vi "main_WS.vi"() -> ()   [LabVIEW 2017]
uses:
  <vilib>/Instr/_visa.llb/VISA Configure Serial Port (Instr).vi
panel:
  out "Waveform Chart":dbl(graph)
  in  "Reconnect":bool
  out "read buffer":string
  in  "Exit":bool
  in  "baud rate":u32=57600
  in  "VISA resource name":refnum<visa-resource-name>="COM1"
  out "tVOC":dbl
  out "CO2":dbl
  out "altitude":dbl
  in  "altitude2":dbl(slide) caption="m" scale=0.0..1000.0 scale format="%#_6p"
  in  "humidity2":dbl(slide) caption="%" scale=0.0..100.0 scale format="%#_6p"
  in  "temperature2":dbl(slide) caption="°C" scale=-20.0..100.0 scale format="%#_6p"
  in  "pressure2":dbl(slide) caption="Pa" scale=110.0..110000.0 scale format="%#_6p"
  out "Humidity":dbl
  out "temperature":dbl
  out "pressure":dbl
  # "Weather Station"
  # "Pressure"
  # "Humidity"
  # "Temperature"
  # "Altitude"
  # "Air quality"
  # "Communication:"
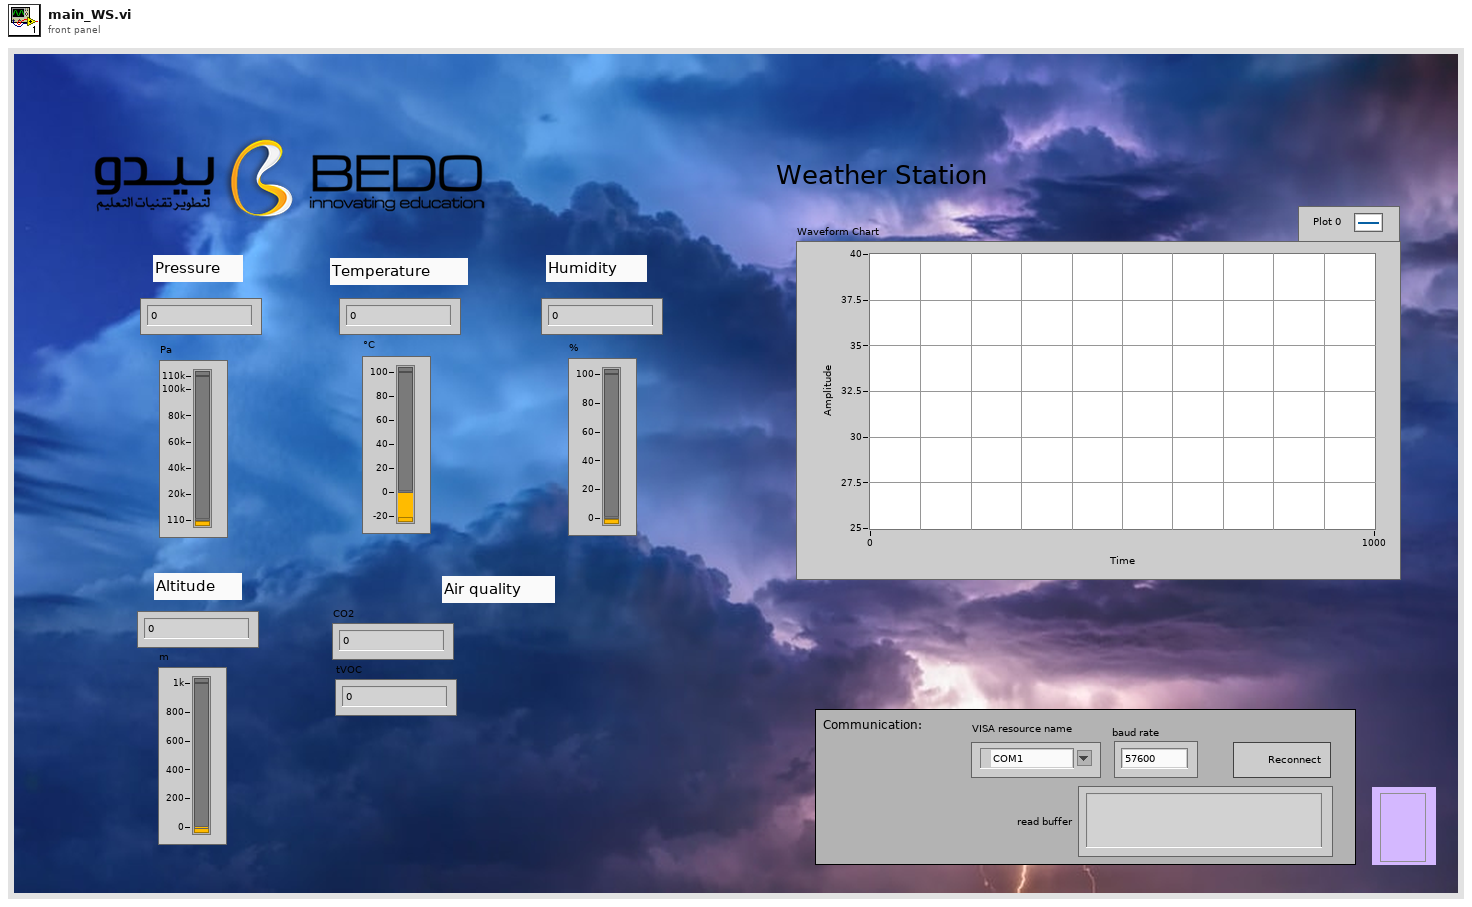
[diagram p1: front panel]
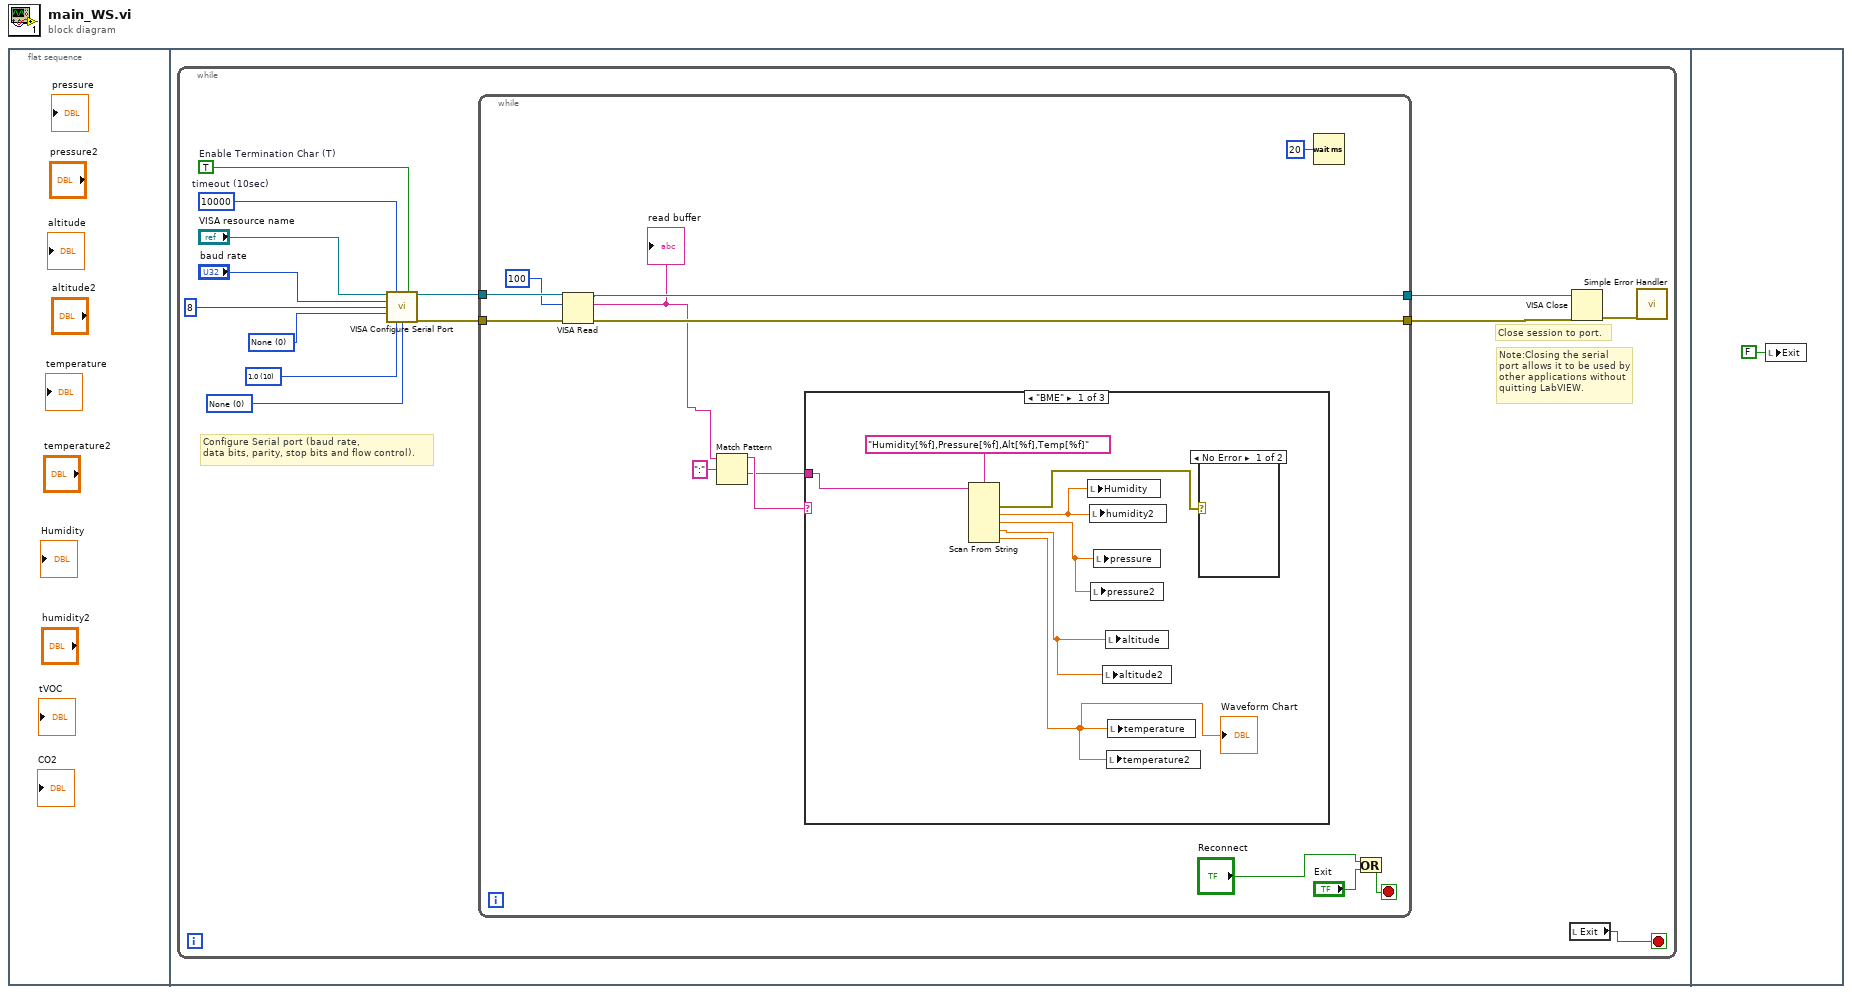
[diagram p0: block diagram]
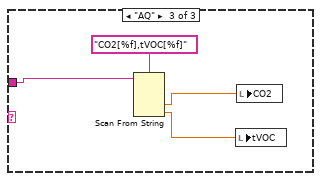
[diagram p4: hidden frame]
diagram:
  n1 = flat-sequence {
    frame #0 {
    }
    frame #1 {
      n2 = while {
        stop <- w1 stop-if-true
        w13 = u16 0 items=["None"=0, "XON/XOFF"=1, "RTS/CTS"=2, "DTR/DSR"=4] ("flow control")
        w12 = u16 10 items=["1.0"=10, "1.5"=15, "2.0"=20] ("stop bits")
        w9 = u16 0 items=["None", "Odd", "Even", "Mark", "Space"] ("parity")
        w11 = TRUE  # Enable Termination Char (T)
        w10 = u32 10000  # timeout (10sec)
        # "Note:Closing the serial port allows it to be used by other applications without\nquitting LabVIEW."
        # "Close session to port."
        # "Configure Serial port (baud rate,\ndata bits, parity, stop bits and flow control)."
        n3 = call-poly "VISA Configure Serial Port"("VISA resource name"="VISA resource name", "timeout (10sec)"=w10, "Enable Termination\nChar (T)"=w11, "baud rate (9600)"="baud rate", "data bits (8)"=u16 8 ("data bits"), "parity (0:none)"=w9, "stop bits (10: 1 bit)"=w12, "flow control (0:none)"=w13) -> ("VISA resource name out"=w6:refnum<visa-resource-name>, "error out"=w5:errorcluster)  [unwired: 6 in]
        n4 = while {
          tunnel: w6 -> [w27]
          tunnel: w5 -> [w26]
          tunnel: [w24] -> w3
          tunnel: [w23] -> w2
          stop <- w15 stop-if-true
          n5 = VISA Read(VISA resource name=w27, byte count=u32 100, error in (no error)=w26) -> (VISA resource name out=w23:refnum<visa-resource-name>, read buffer=w19:string, error out=w24:errorcluster)  [unwired: 1 out]
          "read buffer" <- w19
          n6 = Match Pattern(string=w19, regular expression=":") -> (before substring=w21:string, after substring=w20:string)  [unwired: 1 in, 2 out]
          n7 = case shown="\"BME\"" w21 {
            tunnel: w20 -> [w33 _ w38]
            frame "BME" {
              n8 = Scan From String(format string="Humidity[%f],Pressure[%f],Alt[%f],Temp[%f]", input string=w33) -> (error out=w29:errorcluster, output 1=w32:dbl, output 2=w31:dbl, output 3=w30:dbl, output 4=w28:dbl)  [unwired: 6 in, 2 out]
              "Waveform Chart" <- w28
              n9 = local write "Humidity"(w32) -> ()
              n10 = local write "humidity2"(w32) -> ()
              n11 = local write "pressure2"(w31) -> ()
              n12 = local write "pressure"(w31) -> ()
              n13 = local write "altitude2"(w30) -> ()
              n14 = local write "altitude"(w30) -> ()
              n15 = local write "temperature2"(w28) -> ()
              n16 = local write "temperature"(w28) -> ()
              n17 = case shown="No Error" w29 {
                frame No Error {
                }
                frame Error {
                }
              }
            }
            frame Default {
            }
            frame "AQ" {
              n18 = Scan From String(format string="CO2[%f],tVOC[%f]", input string=w38) -> (output 1=w36:dbl, output 2=w35:dbl)  [unwired: 4 in, 3 out]
              n19 = local write "tVOC"(w35) -> ()
              n20 = local write "CO2"(w36) -> ()
            }
          }
          n21 = Wait (ms)(milliseconds to wait=u32 20) -> ()  [unwired: 1 out]
          n22 = Or(x="Reconnect", y="Exit") -> (x .or. y?=w15:bool)
        }
        n23 = local read "Exit"() -> (w1:bool)
        n24 = VISA Close(VISA resource name=w2, error in (no error)=w3) -> (error out=w4:errorcluster)
        n25 = call <vilib>:"Simple Error Handler.vi"("error in (no error)"=w4) -> ()  [unwired: 4 in, 5 out]
      }
    }
    frame #2 {
      n26 = local write "Exit"(FALSE ("Exit")) -> ()
    }
  }
